vi "Waveform-Create.vi"(6 "Rep Num":i32, 7 "Name":string, 8 "error in (no error)":errorcluster, 9 "Npts":i32, 10 "Sampling Rate (Hz)":dbl, 11 "Waveform":T1={"Type"=enum."Tone", "Tone"={"Frequency (kHz)"=0.0, "Last Freq"=0.0, "Last Phase"=0.0}, "Pulse Train"={"Pulse width (us)"=0.0, "Pulse rate (Hz)"=0.0, "Gap (ms)"=0.0, "Polarity"=enum."POS", "PT State"={"Template"=[], "Nperiod"=0, "Index"=0, "Pulse Rate (Hz)"=0.0, "Phase (cycles)"=0.0, "Noff"=0}, "Asynch"=FALSE}, "Noise"={"InvFilt"=FALSE, "Noise"=[], "CurPt"=0, "Aweight"=FALSE, "Seed"=0, "afile"=path ""}, "File"={"Filename"=path "", "Signal"=[], "Channel"=0, "stream"=FALSE, "offset"=0, "nreps"=0, "loops"=0, "Randomize"=FALSE, "order"=[], "Seed"=0, "Tokens"=0}, "FMSweep"={"Rate (oct/s)"=0.0, "Fmin (Hz)"=0.0, "Fmax (Hz)"=0.0, "Ramp (ms)"=0.0, "Linear"=FALSE}, "Chirp Train"={"Params"={"Fmin (kHz)"=4.0, "Fmax (kHz)"=64.0, "Compensate"=FALSE, "Duration (ms)"=2.0}, "Data"={"WF"=[]}}, "Complex Tone"={"Params"={"F0 (Hz)"=0.0, "Band"={"Flow (Hz)"=0.0, "Fhigh (Hz)"=0.0}, "Phase"=enum."Cosine", "Min F0 (Hz)"=0.0, "Max F0 (Hz)"=0.0, "ContinRandPhase"=FALSE, "Max peak factor"=inf, "Max mod depth"=2.0, "MinHarmNum"=0, "MaxHarmNum"=0, "Level Mode"=enum."per component", "% jitter"=0.0}, "Data"={"Ncomp"=0, "MinHarm"=0, "Phase"=[], "Amplitude"=[], "Npts/frame"=0, "Last F0"=0.0, "Fmin"=0.0, "Fmax"=0.0, "Lslope"=0.0, "randphase"=FALSE, "overall rms"=FALSE, "fmult"=[], "jittered"=FALSE}}, "Moving Ripple"={"Params"={"Fmin"=0.0, "Fmax"=0.0, "Density"=0.0, "Velocity"=0.0, "Depth"=0.0, "Phase"=0.0, "Comp/oct"=0}, "Data"={"Freq"=[], "A"=[], "phase"=[], "Phase"=0.0}}}) -> (0 "error out":errorcluster, 2 "Signal":dbl[](array[numeric]), 3 "Waveform out":T1={"Type"=enum."Tone", "Tone"={"Frequency (kHz)"=0.0, "Last Freq"=0.0, "Last Phase"=0.0}, "Pulse Train"={"Pulse width (us)"=0.0, "Pulse rate (Hz)"=0.0, "Gap (ms)"=0.0, "Polarity"=enum."POS", "PT State"={"Template"=[], "Nperiod"=0, "Index"=0, "Pulse Rate (Hz)"=0.0, "Phase (cycles)"=0.0, "Noff"=0}, "Asynch"=FALSE}, "Noise"={"InvFilt"=FALSE, "Noise"=[], "CurPt"=0, "Aweight"=FALSE, "Seed"=0, "afile"=path ""}, "File"={"Filename"=path "", "Signal"=[], "Channel"=0, "stream"=FALSE, "offset"=0, "nreps"=0, "loops"=0, "Randomize"=FALSE, "order"=[], "Seed"=0, "Tokens"=0}, "FMSweep"={"Rate (oct/s)"=0.0, "Fmin (Hz)"=0.0, "Fmax (Hz)"=0.0, "Ramp (ms)"=0.0, "Linear"=FALSE}, "Chirp Train"={"Params"={"Fmin (kHz)"=4.0, "Fmax (kHz)"=64.0, "Compensate"=FALSE, "Duration (ms)"=2.0}, "Data"={"WF"=[]}}, "Complex Tone"={"Params"={"F0 (Hz)"=0.0, "Band"={"Flow (Hz)"=0.0, "Fhigh (Hz)"=0.0}, "Phase"=enum."Cosine", "Min F0 (Hz)"=0.0, "Max F0 (Hz)"=0.0, "ContinRandPhase"=FALSE, "Max peak factor"=inf, "Max mod depth"=2.0, "MinHarmNum"=0, "MaxHarmNum"=0, "Level Mode"=enum."per component", "% jitter"=0.0}, "Data"={"Ncomp"=0, "MinHarm"=0, "Phase"=[], "Amplitude"=[], "Npts/frame"=0, "Last F0"=0.0, "Fmin"=0.0, "Fmax"=0.0, "Lslope"=0.0, "randphase"=FALSE, "overall rms"=FALSE, "fmult"=[], "jittered"=FALSE}}, "Moving Ripple"={"Params"={"Fmin"=0.0, "Fmax"=0.0, "Density"=0.0, "Velocity"=0.0, "Depth"=0.0, "Phase"=0.0, "Comp/oct"=0}, "Data"={"Freq"=[], "A"=[], "phase"=[], "Phase"=0.0}}})   [LabVIEW 2020]
doc: "Takes a generic waveform description and returns a token of the specific waveform."
uses:
  Controls/Waveform XCtl/Waveform Data.ctl
  Controls/Waveform XCtl/Waveform Enum.ctl
  Tone VIs/Tone Params.ctl
  Pulse Train VIs/Pulse Train Params.ctl
  Pulse Train VIs/Pulse Polarity.ctl
  Pulse Train VIs/PT-Continuous State.ctl
  Noise VIs/Noise Params.ctl
  File VIs/StimFile-Params.ctl
  FM Sweep VIs/FM Sweep Params.ctl
  Chirp Train VIs/Chirp Train.ctl
  Chirp Train VIs/Chirp Train Params.ctl
  Complex Tone VIs/CT-Params.ctl
  Complex Tone VIs/CT-Phase Enum.ctl
  Complex Tone VIs/CT-Runtime Data.ctl
  Moving Ripple VIs/Moving Ripple.ctl
  Moving Ripple VIs/Moving Ripple.Params.ctl
  Moving Ripple VIs/Moving Ripple.Data.ctl
  Controls/Waveform XCtl/Waveform XCtl.xctl
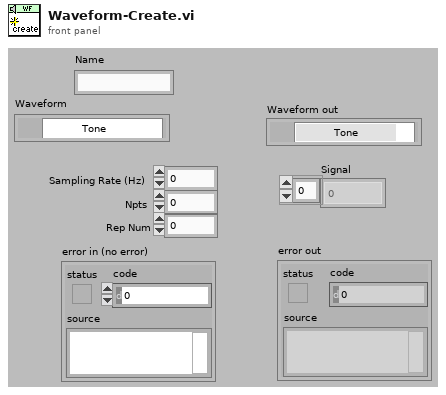
[diagram p1: front panel]
types:
  T1 = typedef "Waveform XCtl.xctl/Waveform Data.ctl" = cluster{"Type":T2, "Tone":T3, "Pulse Train":T4, "Noise":T7, "File":T8, "FMSweep":T9, "Chirp Train":T10, "Complex Tone":cluster{"Params":T12, "Data":T14}, "Moving Ripple":T15}
  T2 = typedef "Waveform Enum.ctl" = enum16{"OFF", "Tone", "Noise", "Pulse Train", "File", "FM Sweep", "Chirp Train", "Complex Tone", "FM Tone", "Moving Ripple"}
  T3 = typedef "Tone Params.ctl" = cluster{"Frequency (kHz)":dbl, "Last Freq":dbl, "Last Phase":dbl}
  T4 = typedef "Pulse Train Params.ctl" = cluster{"Pulse width (us)":dbl, "Pulse rate (Hz)":dbl, "Gap (ms)":dbl, "Polarity":T5, "PT State":T6, "Asynch":bool}
  T5 = typedef "Pulse Polarity.ctl" = enum16{"POS", "NEG", "POS-NEG", "NEG-POS"}
  T6 = typedef "PT-Continuous State.ctl" = cluster{"Template":dbl[], "Nperiod":i32, "Index":i32, "Pulse Rate (Hz)":dbl, "Phase (cycles)":dbl, "Noff":i32}
  T7 = typedef "Noise Params.ctl" = cluster{"InvFilt":bool, "Noise":dbl[], "CurPt":i32, "Aweight":bool, "Seed":i32, "afile":path}
  T8 = typedef "StimFile-Params.ctl" = cluster{"Filename":path, "Signal":dbl[], "Channel":i32, "stream":bool, "offset":i32, "nreps":i32, "loops":i32, "Randomize":bool, "order":i32[], "Seed":i32, "Tokens":i32}
  T9 = typedef "FM Sweep Params.ctl" = cluster{"Rate (oct/s)":dbl, "Fmin (Hz)":dbl, "Fmax (Hz)":dbl, "Ramp (ms)":dbl, "Linear":bool}
  T10 = typedef "Chirp Train.ctl" = cluster{"Params":T11, "Data":cluster{"WF":dbl[]}}
  T11 = typedef "Chirp Train Params.ctl" = cluster{"Fmin (kHz)":dbl, "Fmax (kHz)":dbl, "Compensate":bool, "Duration (ms)":dbl}
  T12 = typedef "CT-Params.ctl" = cluster{"F0 (Hz)":dbl, "Band":cluster{"Flow (Hz)":dbl, "Fhigh (Hz)":dbl}, "Phase":T13, "Min F0 (Hz)":dbl, "Max F0 (Hz)":dbl, "ContinRandPhase":bool, "Max peak factor":dbl, "Max mod depth":dbl, "MinHarmNum":i32, "MaxHarmNum":i32, "Level Mode":enum16{"per component", "overall rms"}, "% jitter":dbl}
  T13 = typedef "CT-Phase Enum.ctl" = enum16{"Cosine", "Random", "Alternating"}
  T14 = typedef "CT-Runtime Data.ctl" = cluster{"Ncomp":i32, "MinHarm":i32, "Phase":dbl[], "Amplitude":dbl[], "Npts/frame":i32, "Last F0":dbl, "Fmin":dbl, "Fmax":dbl, "Lslope":dbl, "randphase":bool, "overall rms":bool, "fmult":dbl[], "jittered":bool}
  T15 = typedef "Moving Ripple.ctl" = cluster{"Params":T16, "Data":T17}
  T16 = typedef "Moving Ripple.Params.ctl" = cluster{"Fmin":dbl, "Fmax":dbl, "Density":dbl, "Velocity":dbl, "Depth":dbl, "Phase":dbl, "Comp/oct":i32}
  T17 = typedef "Moving Ripple.Data.ctl" = cluster{"Freq":dbl[], "A":dbl[], "phase":dbl[], "Phase":dbl}
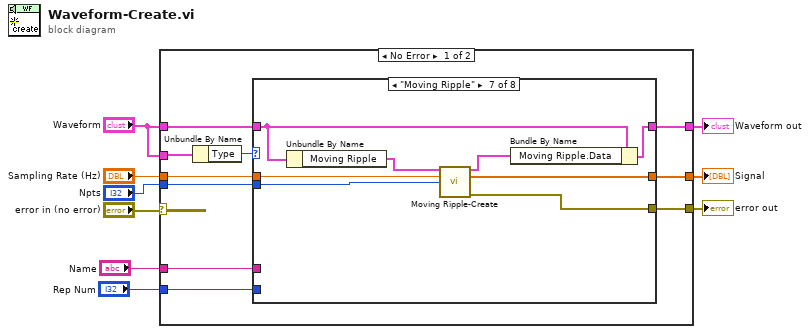
[diagram p0: block diagram]
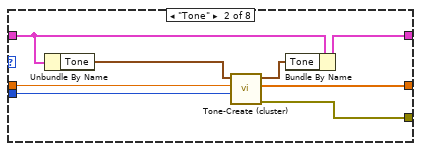
[diagram p3: hidden frame]
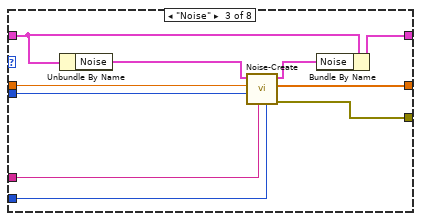
[diagram p4: hidden frame]
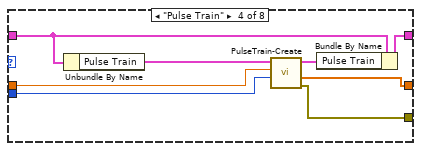
[diagram p5: hidden frame]
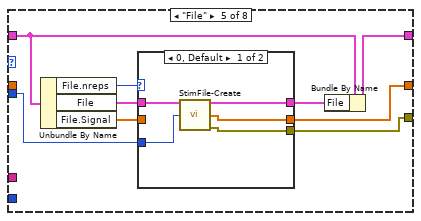
[diagram p6: hidden frame]
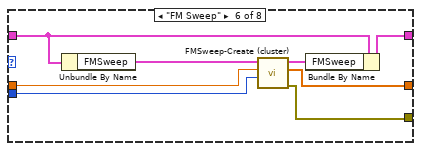
[diagram p8: hidden frame]
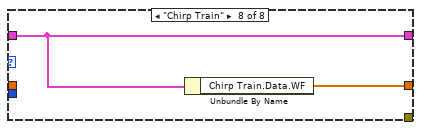
[diagram p9: hidden frame]
diagram:
  n1 = case shown="No Error" "error in (no error)" {
    selector: "error in (no error)" -> [_ w82]
    tunnel: [w14 w82] -> w8
    tunnel: "Waveform" -> [w19 _]
    tunnel: "Sampling Rate (Hz)" -> [w17 _]
    tunnel: "Npts" -> [w16 _]
    tunnel: "Waveform" -> [w15 w81]
    tunnel: [w13 _] -> w4
    tunnel: [w12 w81] -> w3
    tunnel: "Name" -> [w11 _]
    tunnel: "Rep Num" -> [w10 _]
    frame No Error {
      n2 = Unbundle By Name(w19) -> ("Type"=w18:T2)
      n3 = case shown="\"Moving Ripple\"" w18 {
        tunnel: w17 -> [_ w28 w38 w44 _ w64 w76 _]
        tunnel: w16 -> [_ w27 w37 w43 w48 w63 w75 _]
        tunnel: w15 -> [w20 w26 w35 w46 w55 w70 w78 w80]
        tunnel: [_ w25 w33 w42 w47 w66 w71 _] -> w14
        tunnel: [_ w24 w32 w41 w50 w65 w72 w79] -> w13
        tunnel: [w20 w23 w31 w40 w52 w68 w77 w80] -> w12
        tunnel: w11 -> [_ _ w30 _ _ _ _ _]
        tunnel: w10 -> [_ _ w29 _ _ _ _ _]
        frame "OFF", Default {
        }
        frame "Tone" {
          n4 = Unbundle By Name(w26) -> ("Tone"=w22:T3)
          n5 = call "Tone-Create (cluster).vi"("Npts"=w27, "Sampling Rate (Hz)"=w28, "Tone Class in"=w22) -> ("error out"=w25:errorcluster, "Waveform"=w24:dbl[], "Tone Class out"=w21:T3)  [unwired: 6 in]
          n6 = Bundle By Name(cluster=w26, "Tone"=w21) -> (w23:T1)
        }
        frame "Noise" {
          n7 = Unbundle By Name(w35) -> ("Noise"=w36:T7)
          n8 = call "Noise-Create.vi"("Rep Num"=w29, "Name"=w30, "Npts"=w37, "Sampling Rate (Hz)"=w38, "Noise Params"=w36) -> ("error out"=w33:errorcluster, "Waveform"=w32:dbl[], "Noise Params (out)"=w34:T7)  [unwired: 4 in]
          n9 = Bundle By Name(cluster=w35, "Noise"=w34) -> (w31:T1)
        }
        frame "Pulse Train" {
          n10 = Unbundle By Name(w46) -> ("Pulse Train"=w45:T4)
          n11 = call "PulseTrain-Create.vi"("Npts"=w43, "Sampling Rate (Hz)"=w44, "Pulse Train Params"=w45) -> ("error out"=w42:errorcluster, "Waveform"=w41:dbl[], "Pulse Train Params (out)"=w39:T4)  [unwired: 5 in, 1 out]
          n12 = Bundle By Name(cluster=w46, "Pulse Train"=w39) -> (w40:T1)
        }
        frame "File" {
          n13 = Unbundle By Name(w55) -> ("File.nreps"=w54:i32, "File"=w53:T8, "File.Signal"=w49:dbl[])
          n14 = case shown="0, Default" w54 {
            tunnel: w53 -> [w60 w62]
            tunnel: [w59 w62] -> w51
            tunnel: [w58 w61] -> w50
            tunnel: w49 -> [_ w61]
            tunnel: w48 -> [w57 _]
            tunnel: [w56 _] -> w47
            frame 0, Default {
              n15 = call "StimFile-Create.vi"("File"=w60, "Npts"=w57) -> ("File out"=w59:T8, "Y"=w58:dbl[], "error out"=w56:errorcluster)  [unwired: 11 in]
            }
            frame 1 {
            }
          }
          n16 = Bundle By Name(cluster=w55, "File"=w51) -> (w52:T1)
        }
        frame "FM Sweep" {
          n17 = Unbundle By Name(w70) -> ("FMSweep"=w69:T9)
          n18 = call "FMSweep-Create (cluster).vi"("Npts"=w63, "Sampling Rate (Hz)"=w64, "FMSweep In"=w69) -> ("error out"=w66:errorcluster, "Waveform"=w65:dbl[], "FMSweep Out"=w67:T9)  [unwired: 6 in]
          n19 = Bundle By Name(cluster=w70, "FMSweep"=w67) -> (w68:T1)
        }
        frame "Moving Ripple" {
          n20 = Unbundle By Name(w78) -> ("Moving Ripple"=w74:T15)
          n21 = call "Moving Ripple-Create.vi"("Moving Ripple"=w74, "Sampling Rate (Hz)"=w76, "Npts"=w75) -> ("Data"=w73:T17, "Array"=w72:dbl[], "error out"=w71:errorcluster)  [unwired: 10 in]
          n22 = Bundle By Name(cluster=w78, "Moving Ripple.Data"=w73) -> (w77:T1)
        }
        frame "Chirp Train" {
          n23 = Unbundle By Name(w80) -> ("Chirp Train.Data.WF"=w79:dbl[])
        }
      }
    }
    frame Error {
    }
  }
  "error out" <- w8
  "Signal" <- w4
  "Waveform out" <- w3
